vi "RH Tester.vi"() -> ()   [LabVIEW 2016]
uses:
  <vilib>/Platform/TimedLoop/XDataNode/timing_clust.ctl
  <vilib>/Platform/TimedLoop/XDataNode/nitl_modes.ctl
  <vilib>/Platform/TimedLoop/XDataNode/wakeup.ctl
  <vilib>/Utility/file.llb/Write To Spreadsheet File (string).vi
  <vilib>/Platform/TimedLoop/XDataNode/XDataNode.xnode
  <vilib>/Platform/TimedLoop/XDataNode/XDNodeRunTimeDep.lvlib
panel:
  out "Probe 2 RH":dbl
  out "Probe 2 (F)":dbl
  in  "Probe 2":string="192.168.1.42"
  out "Probe 1 RH":dbl
  out "Probe 1 (F)":dbl
  in  "Probe 1":string="192.168.1.41"
  in  "Chamber Temp":string="192.168.1.161"
  in  "Log Data":bool
  out "RH":cluster{dbl[], dbl[]}[](graph)
  in  "Period(s)":i32=1
  in  "Max Num to Chart":i32=1000
  out "Temp":cluster{dbl[], dbl[]}[](graph)
  out "Chamber RH":dbl
  out "Chamber Temp (F)":dbl
  out "time stamp":timestamp
  out "Count":i32
  in  "stop":bool
  in  "file path (dialog if empty)":path=path "c:/data/RH_Log_Data.csv"
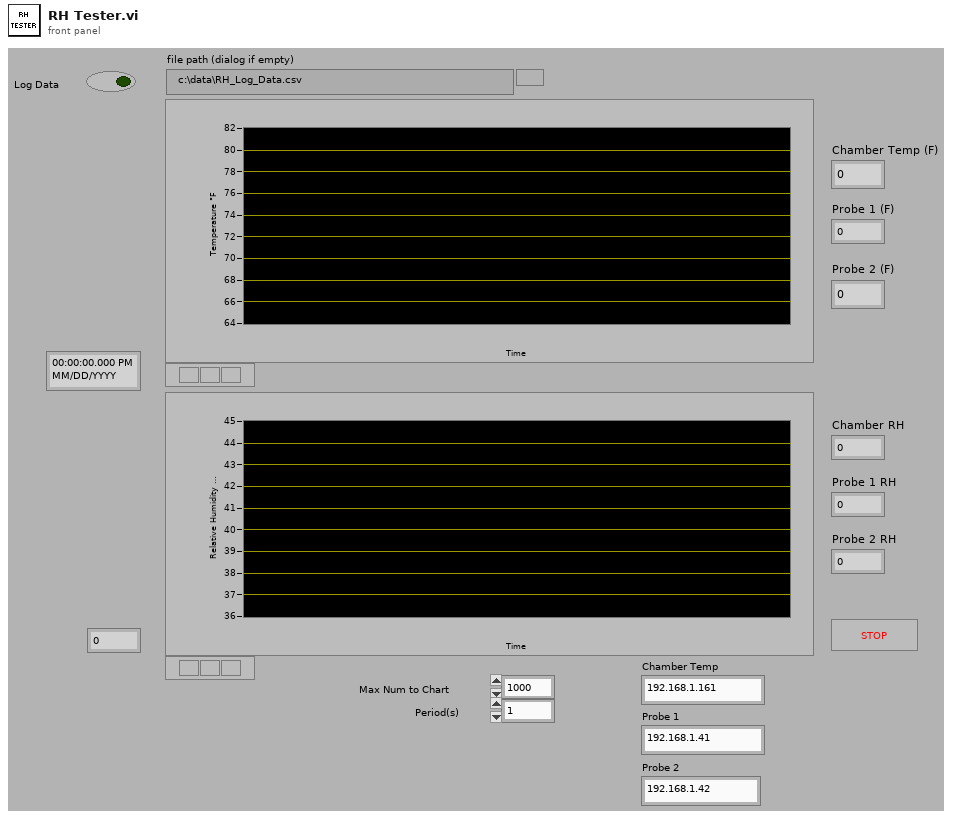
[diagram p1: front panel]
types:
  T1 = typedef "XDNodeRunTimeDep.lvlib/timing_clust.ctl" = cluster{"Expected End [f-1]":u64, "Actual End [f-1]":u64, "Finished Late? [f-1]":bool, "Expected End [i-1]":u64, "Actual End [i-1]":u64, "Finished Late? [i-1]":bool, "Expected Start [i]":u64, "Actual Start [i]":u64, "Expected Start [f]":u64, "Actual Start [f]":u64, "Source Name":string, "Structure Name":string, "Period":i64, "Deadline":i64, "Offset":i64, "Start":i64, "Priority":i32, "Timeout":i32, "Mode":T2, "Wakeup Reason":T3, "Error":errorcluster, "Source Type":string, "Secondary Source Type":string, "Global End Time":u64, "Global Start Time":u64, "Frame Duration":u64, "Iteration Duration":u64, "Assigned CPU":i32, "I/O Scan Engine Mode":u32}
  T2 = typedef "XDNodeRunTimeDep.lvlib/nitl_modes.ctl" = enum32{"No Change", "Process missed periods, maintain original phase", "Discard missed periods, maintain original phase", "Process missed periods, ignore original phase", "Discard missed periods, ignore original phase"}
  T3 = typedef "XDNodeRunTimeDep.lvlib/wakeup.ctl" = enum32{"Normal", "Aborted", "Asynchronous wakeup", "Timing source error", "Timed loop error", "Timeout"}
  T4 = typedef "iBTHX Data Values.ctl" = cluster{"iBTHX Barometric Pressure (mbar/hPa)":dbl, "iBTHX Humidity (%)":dbl, "iBTHX Temperature (°F)":dbl, "iBTHX DewPoint Temp":dbl}
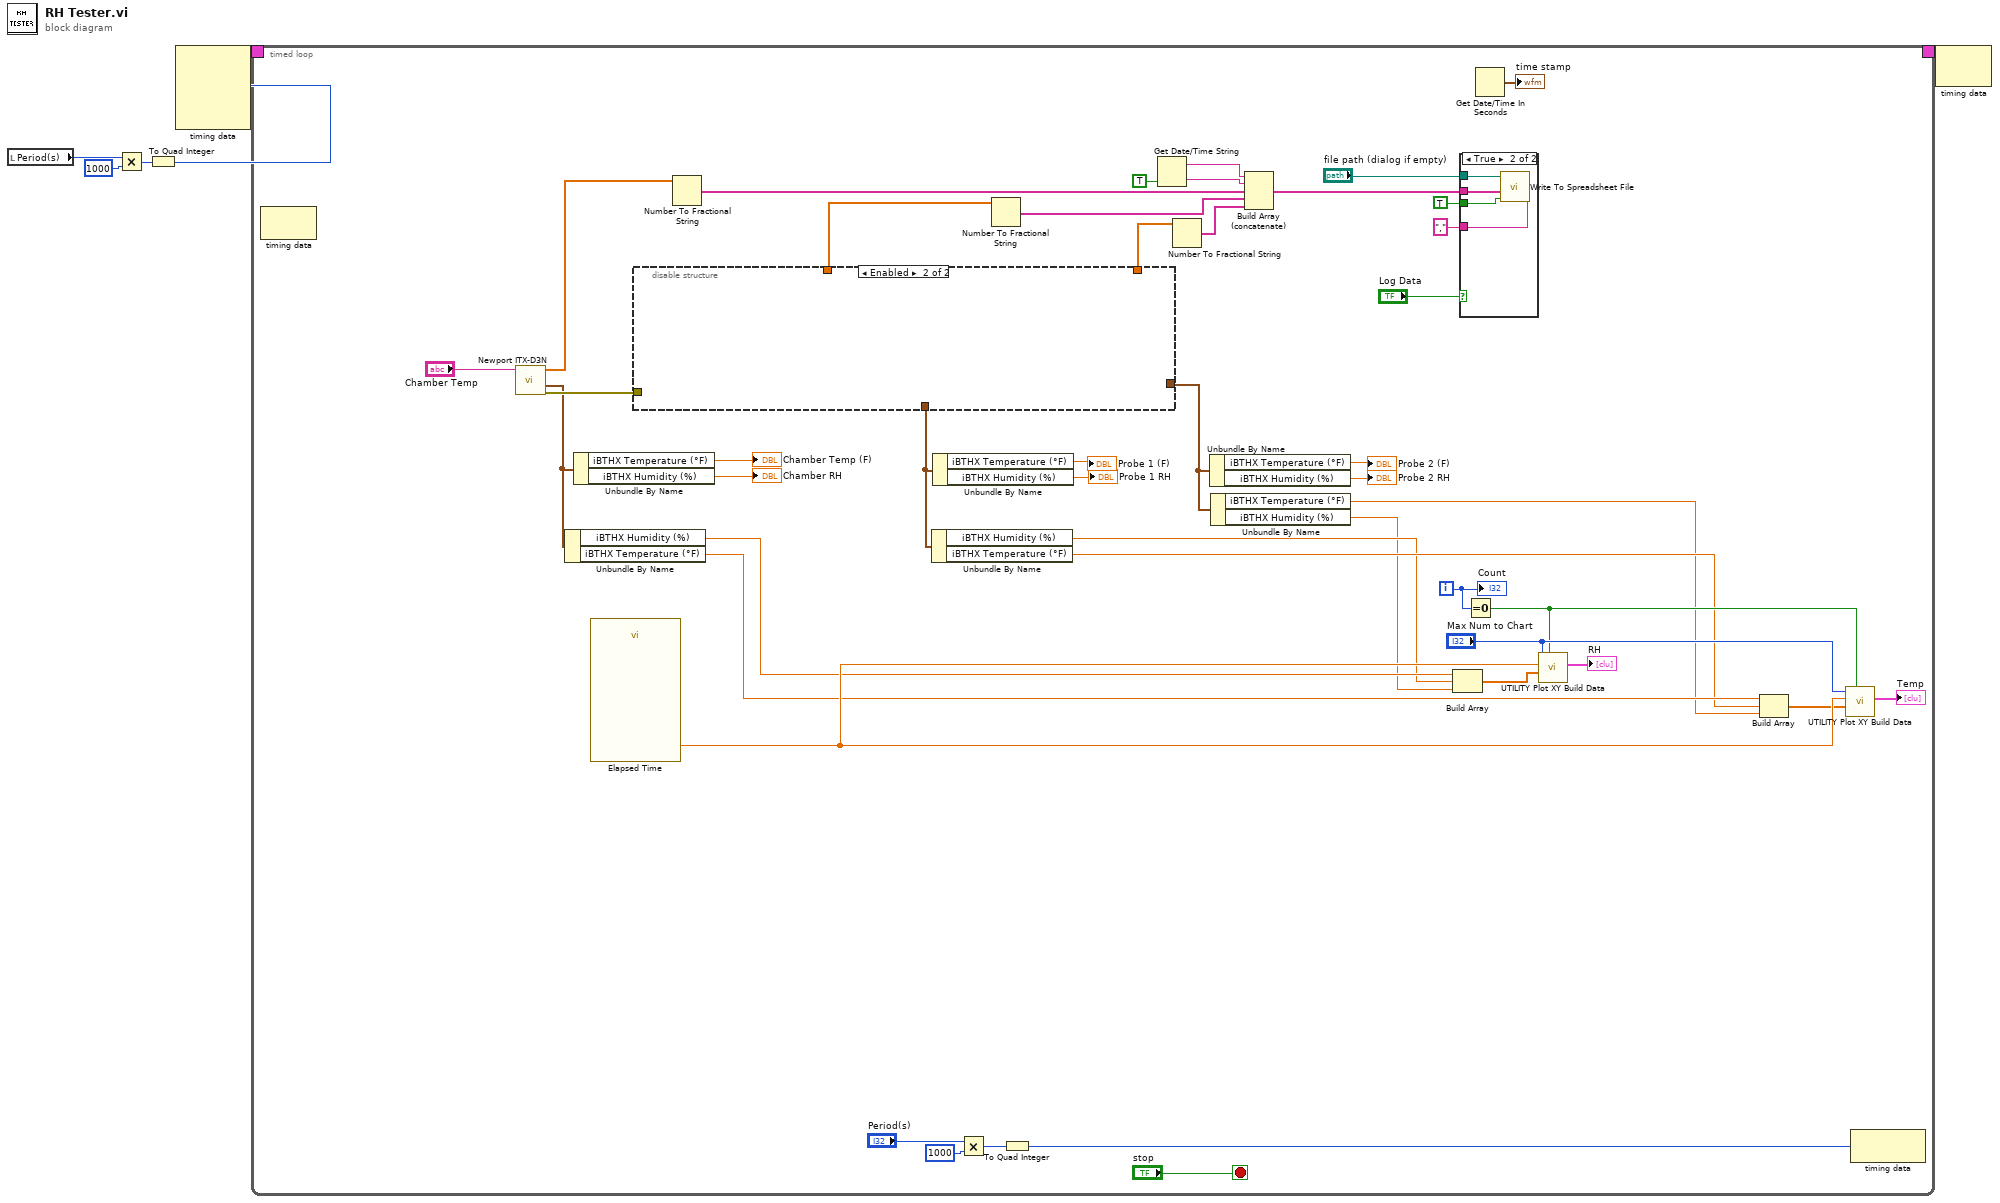
[diagram p0: block diagram]
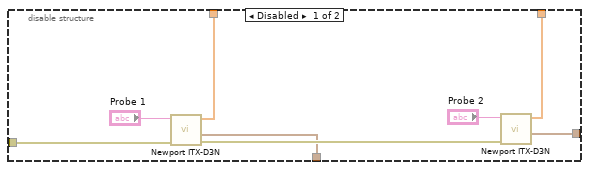
[diagram p2: hidden frame]
diagram:
  n1 = local read "Period(s)"() -> (w1:i32)
  n2 = Multiply(x=w1, y=1000) -> (x*y=w3:i32)
  n3 = To Quad Integer(1:w3) -> (0:w2:i64)
  n4 = node-c288(w2) -> (w6:T1)  [unwired: 3 in]
  n5 = timed-loop {
    timing: w6 -> [_]
    timing-out: [_] -> w5
    i -> [w33]
    stop <- "stop" stop-if-true
    n6 = node-c288() -> ()  [unwired: 1 in, 1 out]
    n7 = call "Newport ITX-D3N.vi"("Machine"="Chamber Temp") -> ("error out"=w23:errorcluster, "iTHX/iBTHX Output"=w9:T4, "Temp/Humidity"=w39:dbl[])  [unwired: 7 in, 1 out]
    n8 = Unbundle By Name(w9) -> ("iBTHX Humidity (%)"=w19:dbl, "iBTHX Temperature (°F)"=w20:dbl)
    n9 = Unbundle By Name(w9) -> ("iBTHX Temperature (°F)"=→"Chamber Temp (F)":dbl, "iBTHX Humidity (%)"=→"Chamber RH":dbl)
    n10 = call "Elapsed Time"() -> ("Present (s)"=w37:dbl)  [unwired: 12 in, 7 out]
    n11 = disable-structure shown="Enabled" {
      disable-tunnel: [w58 _] -> w26
      disable-tunnel: [w56 _] -> w25
      disable-tunnel: w23 -> [w55 _]
      disable-tunnel: [w53 _] -> w8
      disable-tunnel: [w52 _] -> w7
      frame Disabled {
        n12 = call "Newport ITX-D3N.vi"("error in (no error)"=w55, "Machine"="Probe 1") -> ("error out"=w54:errorcluster, "iTHX/iBTHX Output"=w53:T4, "Temp/Humidity"=w58:dbl[])  [unwired: 6 in, 1 out]
        n13 = call "Newport ITX-D3N.vi"("error in (no error)"=w54, "Machine"="Probe 2") -> ("iTHX/iBTHX Output"=w52:T4, "Temp/Humidity"=w56:dbl[])  [unwired: 6 in, 2 out]
      }
      frame Enabled {
      }
    }
    n14 = Number To Fractional String(number=w39) -> (F-format string=w47:string[])  [unwired: 3 in]
    n15 = Unbundle By Name(w8) -> ("iBTHX Humidity (%)"=w14:dbl, "iBTHX Temperature (°F)"=w15:dbl)
    n16 = Unbundle By Name(w8) -> ("iBTHX Temperature (°F)"=→"Probe 1 (F)":dbl, "iBTHX Humidity (%)"=→"Probe 1 RH":dbl)
    n17 = Multiply(x="Period(s)", y=1000) -> (x*y=w31:i32)
    n18 = Number To Fractional String(number=w26) -> (F-format string=w27:string[])  [unwired: 3 in]
    n19 = To Quad Integer(1:w31) -> (0:w29:i64)
    n20 = Get Date/Time String(want seconds? (F)=TRUE) -> (date string=w49:string, time string=w48:string)  [unwired: 2 in]
    n21 = Number To Fractional String(number=w25) -> (F-format string=w18:string[])  [unwired: 3 in]
    n22 = Unbundle By Name(w7) -> ("iBTHX Temperature (°F)"=→"Probe 2 (F)":dbl, "iBTHX Humidity (%)"=→"Probe 2 RH":dbl)
    n23 = Unbundle By Name(w7) -> ("iBTHX Temperature (°F)"=w11:dbl, "iBTHX Humidity (%)"=w10:dbl)
    n24 = Build Array (concatenate)(w49, w48, w47, w27, w18) -> (w45:string[])
    n25 = Build Array(w19, w14, w10) -> (w36:dbl[])
    n26 = case shown="True" "Log Data" {
      tunnel: "file path (dialog if empty)" -> [_ w63]
      tunnel: w45 -> [_ w62]
      tunnel: TRUE ("append to file? (new file:F)") -> [_ w61]
      tunnel: "," ("delimiter (\\t)") -> [_ w60]
      frame False {
      }
      frame True {
        n27 = call-poly <vilib>:"Write To Spreadsheet File.vi"("delimiter (\\t)"=w60, "append to file? (new file:F)"=w61, "1D data"=w62, "file path (dialog if empty)"=w63) -> ()  [unwired: 4 in, 1 out]
      }
    }
    n28 = Equal To 0?(x=w33) -> (x = 0?=w32:bool)
    n29 = Get Date/Time In Seconds() -> (seconds since 1Jan1904=→"time stamp":timestamp)
    n30 = call "UTILITY Plot XY Build Data.vi"("Reset"=w32, "Data Array"=w36, "Time (s)"=w37, "Max Array Size"="Max Num to Chart") -> ("Plot Data"=→"RH":cluster{dbl[], dbl[]}[])  [unwired: 7 in]
    n31 = Build Array(w20, w15, w11) -> (w35:dbl[])
    n32 = call "UTILITY Plot XY Build Data.vi"("Reset"=w32, "Data Array"=w35, "Time (s)"=w37, "Max Array Size"="Max Num to Chart") -> ("Plot Data"=→"Temp":cluster{dbl[], dbl[]}[])  [unwired: 7 in]
    n33 = node-c288(w29) -> ()  [unwired: 1 out]
    "Count" <- w33
  }
  n34 = node-c288(w5) -> ()  [unwired: 1 out]
